vi "SP Read Single.vi"(8 "error in":errorcluster, 9 "Channel Index":i32=1, 11 "Temperature Setpoint in":refnum<class "Temperature Setpoint.lvclass">) -> (0 "error out":errorcluster, 1 "Changed or First Call?":bool, 2 "Temperature SP":dbl, 3 "Temperature Setpoint out":refnum<class "Temperature Setpoint.lvclass">)   [LabVIEW 2023, in "Temperature Setpoint.lvclass"]
uses:
  Temperature Setpoint.lvclass
  Parents/Setpoint/Setpoint.lvclass
  Temperature Setpoint.lvclass/Temperature Setpoint.ctl
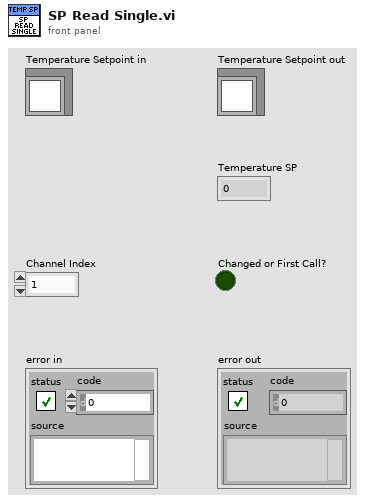
[diagram p1: front panel]
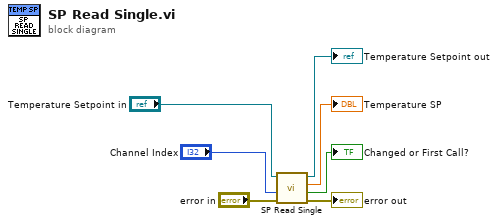
[diagram p0: block diagram]
diagram:
  n1 = call-parent "SP Read Single.vi"("error in"="error in", "Channel Index"="Channel Index", "Setpoint in"="Temperature Setpoint in") -> ("error out"=→"error out":errorcluster, "Changed or First Call?"=→"Changed or First Call?":bool, "Current SP"=→"Temperature SP":dbl, "Setpoint out"=→"Temperature Setpoint out":refnum<class "Temperature Setpoint.lvclass">)  [unwired: 5 in]
